vi "JSONRPC Server.vi"(7 "LabVIEW Web Service":refnum<class "Web Service.lvclass">) -> ()   [LabVIEW 2017]
uses:
  <vilib>/wsapi/Web Service.lvclass
  <vilib>/NI/NI JSONRPC Server Framework/Classes/Server/JSONRPC Server.lvclass
panel:
  in  "error in (no error)":errorcluster
  out "error out":errorcluster
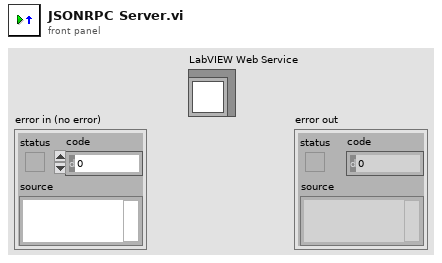
[diagram p1: front panel]
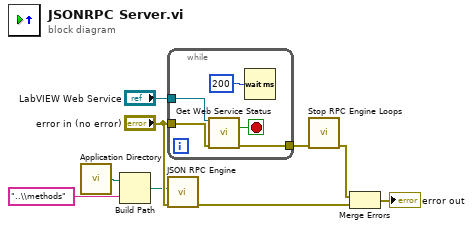
[diagram p0: block diagram]
diagram:
  n1 = call <vilib>:"Application Directory.vi"() -> ("Application Directory"=w3:path)
  n2 = Build Path(base path=w3, name or relative path="..\\methods") -> (appended path=w1:path)
  n3 = while {
    tunnel: [w13] -> w9
    tunnel: "error in (no error)" -> [w12]
    tunnel: "LabVIEW Web Service" -> [w11]
    stop <- w14 stop-if-true
    n4 = call <vilib>:"Get Web Service Status.vi"("LabVIEW Web Service"=w11, "error in (no error)"=w12) -> ("service stopping?"=w14:bool, "error out"=w13:errorcluster)  [unwired: 11 in, 1 out]
    n5 = Wait (ms)(milliseconds to wait=u32 200) -> ()  [unwired: 1 out]
  }
  n6 = call <vilib>:"JSON RPC Engine.vi"("error in (no error)"="error in (no error)", "methods directory"=w1) -> ("error out"=w4:errorcluster)  [unwired: 9 in]
  n7 = call <vilib>:"Stop RPC Engine Loops.vi"("error in (no error)"=w9) -> ("error out"=w6:errorcluster)  [unwired: 10 in]
  n8 = Merge Errors(w6, w4) -> (→"error out":errorcluster)
